vi "set_technique_sequence.vi"(3 "input_machine_reference.lvclass":refnum<class "machine.lvclass">) -> (1 "output_machine_reference.lvclass":refnum<class "machine.lvclass">)   [LabVIEW 2014, in "machine.lvclass"]
uses:
  machine.lvclass
  machine.lvclass/machine.ctl
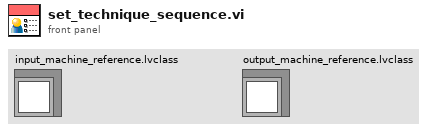
[diagram p1: front panel]
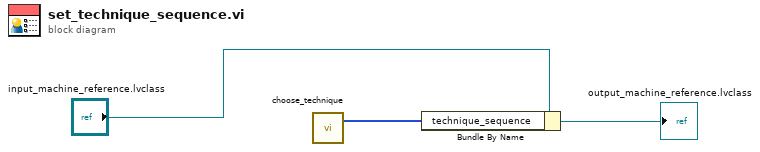
[diagram p0: block diagram]
diagram:
  n1 = call "choose_technique.vi"() -> ("technique_sequence"=w1:i32[])  [unwired: 3 in]
  n2 = Bundle By Name(cluster="input_machine_reference.lvclass", "technique_sequence"=w1) -> (→"output_machine_reference.lvclass":refnum<class "machine.lvclass">)
